vi "UHR-Fleezers Control (host) - Lorentz v4.vi"() -> ()   [LabVIEW 2014] (continued)
  in  "Chemyx Syringe Pump Serial Port":refnum<visa-resource-name>="ASRL3::INSTR"
  in  "Limit Min (MHz)":dbl=10.0 caption="Min (MHz)"
  in  "Limit Max (MHz)":dbl=16.0 caption="Max (MHz)"
  in  "Limits Enable":bool=TRUE caption="Enable"
  out "AI labels":string[](array[string])=["T1 Y", "T1 X", "T1 Sum", "T2 Y", "T2 X", "T2 Sum", "T1 FB X", "T1 FB Sum", "T2 FB X", "T2 FB Sum", "T3 Y", "T3 X", "T3 Sum", "PSD X", "PSD Y", "PSD Sum"]
  in  "Save Trap Pos. Data":bool=TRUE
  in  "Lower Ch. Cap.":bool
  in  "Top 3 Harvard Syringe Pump Serial Port":refnum<visa-resource-name>="Top-Pump3-COM4"
  out "Database link":path=path "C:/Home/Bustamante Lab/Comstock-LabView-Link.udl"
  out "connection reference":T25
  out "FPGA error out":errorcluster
  out "Trigger Signal":dbl[](graph)=[1.953852737276498, 1.8613052147403675]
  in  "Fish mask thresh":dbl=0.5
  in  "Normal (on) or masked test (off)":bool=TRUE
  in  "Stop F (pN) (mask)":dbl=1.0
  in  "Osc. freq. (Hz)":dbl=0.25
  in  "Trap shift\nmethod":bool=TRUE
  in  "Pause rotation":bool
  out "Waveform Chart":dbl(graph)
  in  "Trap 2 phase shift (deg)":dbl caption="Fixed phase shift (deg)"
  in  "Radius (MHz)":dbl=2.0 min=0.0 max=10.0 step=0.1
  out "Trap trajectories":cluster{dbl[], dbl[]}[](graph)
  in  "Move in a Circle":bool
  in  "Center Y Frequency (MHz)":dbl=31.0
  in  "Stop Moving":bool
  in  "2D Motion Frequency (Hz)":dbl=0.25
  in  "2D Motion Trap Separation (MHz)":dbl=0.75 caption="Fixed distance (MHz)" min=0.0 max=10.0 step=0.1
  in  "Time step (ms)":i64=10
  in  "N steps then stop":i32
  in  "Back to start on finish?":bool=TRUE
  in  "Counterclockwise/Clockwise":bool
  out "Trap 1 sum mean":dbl=nan format="%0.2f"
  out "Trap 2 sum mean":dbl=nan format="%0.2f"
  in  "index 1":i32=3
  in  "index 2":i32
  in  "test":bool
  in  "Reset graph":bool
  in  "N steps to plot":i32=1000
  out "Waveform Graph 2":waveform(dbl)(graph)
  in  "Offset 2":dbl
  in  "mult x":dbl
  in  "Offset":dbl
  out "N data samples":dbl
  out "Initial buffer time (s)":dbl
  in  "N initial buffer elements":u16=5000
  in  "Sound ON":bool
  in  "Carrier Frequency (Hz)":dbl=300.0
  in  "number of samples/ch":i32=100000
  in  "sample mode":T26=1 items=["Finite Samples", "Continuous Samples"]
  in  "device ID":u32
  in  "sound format":T27={"sample rate (S/s)"=22050.0, "number of channels"=2, "bits per sample"=16}
  in  "Volume":dbl=1.0 format="%0.2p"
  in  "interpolation mode":u16(ring)=1 items=["coerce", "linear", "spline", "FIR filter"]
  in  "tone or data":bool
  in  "Data channel to sound":i32
  in  "Base N trap periods":u32=50
  in  "Period scale factor":dbl=4.0
  in  "Trap osc amp (MHz)":dbl=1.0
  in  "Osc trap cont.":bool
  in  "Osc traps":bool
  out "Trap OSC Period (s)":dbl=0.003
  out "Writing waveform to fpga memory":bool
  in  "Save trap pos with cal":bool=TRUE
  in  "T1 Osc Enable":bool=TRUE
  in  "T2 Osc Enable":bool=TRUE
  out "DMA remainder":u64
  out "(total save/100) /osc period remainder":u32
  out "Total save/100 remainder":u32
  out "N osc/ (total save/100)":u64=25
  out "N osc / DMA":u64=100
  out "N trap osc periods per save":u64
  out "N trap osc periods per save remainder":u64
  in  "Command":string
  out "Reply":string
  in  "Send Command":bool
  out "Preamp Error Out":errorcluster
  in  "Gain Mode":string(combo)="0"
  in  "Invert Signal":bool
  in  "Sensitivity":string(combo)="0"
  in  "Offset Current Sign":bool=TRUE
  in  "Offset Current Value":string(combo)
  in  "Offset Current":bool
  in  "Bias Voltage":bool
  in  "Bias Voltage (mV)":i32
  in  "Filter Type":string(combo)="4"
  in  "Lowpass 3dB Point":string(combo)="6"
  in  "Highpass 3dB Point":string(combo)
  in  "Filter Reset":bool
  out "Command Sent":string
  out "Gain":string(combo)="0"
  out "Pressure":dbl=0.014364525990046895 format="%#.2f"
  in  "Vacuum":bool=TRUE
  in  "Set zero pressure":bool caption="Vent pressure"
  in  "DAQmx Device Name":tag="Lumicks"
  out "Channel 3":T28={"X Pos (mm)"=0.15566698, "Y Pos (mm)"=-0.21665113, "Z Pos (mm)"=-0.11814949} {"Y Pos (mm)" format="%.3f"; "Z Pos (mm)" format="%.3f"; "X Pos (mm)" format="%.3f"}
  out "Channel 2":T28={"X Pos (mm)"=0.39374417, "Y Pos (mm)"=-0.0075209886, "Z Pos (mm)"=-0.07494753} {"Y Pos (mm)" format="%.3f"; "Z Pos (mm)" format="%.3f"; "X Pos (mm)" format="%.3f"}
  out "Channel 1":T28={"X Pos (mm)"=-1.904501, "Y Pos (mm)"=-0.42059234, "Z Pos (mm)"=-0.07494753} {"Y Pos (mm)" format="%.3f"; "Z Pos (mm)" format="%.3f"; "X Pos (mm)" format="%.3f"}
  in  "Motor Cruise Param":T29={"Y Acc (mm/s^2)"=0.1, "Y Vmax (mm/s)"=1.0, "X Acc (mm/s^2)"=0.3, "X Vmax (mm/s)"=1.0, "Z Acc (mm/s^2)"=0.1, "Z Vmax (mm/s)"=0.1}
  out "Channel 4":T28={"X Pos (mm)"=-2.403743, "Y Pos (mm)"=0.10211637, "Z Pos (mm)"=-0.074918374} {"Y Pos (mm)" format="%.3f"; "Z Pos (mm)" format="%.3f"; "X Pos (mm)" format="%.3f"}
  out "0 Position":T28 {"Y Pos (mm)" format="%.3f"; "Z Pos (mm)" format="%.3f"; "X Pos (mm)" format="%.3f"}
  in  "Calibration Cruise Param":T29={"Y Acc (mm/s^2)"=2.0, "Y Vmax (mm/s)"=0.5, "X Acc (mm/s^2)"=2.0, "X Vmax (mm/s)"=0.5, "Z Acc (mm/s^2)"=0.1, "Z Vmax (mm/s)"=0.1}
  in  "Read Coordinates":bool
  in  "Write Coordinates":bool
  in  "4-Experiment position":bool
  in  "Capture Channel 4":bool
  out "Channel 5":T28={"X Pos (mm)"=0.15566698, "Y Pos (mm)"=-0.2807253, "Z Pos (mm)"=-0.118062034} {"Y Pos (mm)" format="%.3f"; "Z Pos (mm)" format="%.3f"; "X Pos (mm)" format="%.3f"}
  in  "Motor settings (Z)":cluster{"Vmax (mm/s)":sgl, "Acc (mm/s/s)":sgl}={"Vmax (mm/s)"=0.02, "Acc (mm/s/s)"=0.2}
  in  "Motor settings (X,Y)":cluster{"Vmax (mm/s)":sgl, "Acc (mm/s/s)":sgl}={"Vmax (mm/s)"=0.2, "Acc (mm/s/s)"=0.2}
  in  "Motor Limits":T30={"XMAX"=3.5, "XMIN"=-5.0, "YMAX"=2.0, "YMIN"=-2.0, "ZMAX"=2.0, "ZMIN"=-2.0}
  out "XYZ position":sgl[](array[numeric])=[0.3568097, 0.022271454, -0.22568797]
  in  "Go to 0 at stop?":bool
  in  "Write Coordinates path":path=path "C:/Data/Coordinates"
  in  "Read Coordinates path":path=path "C:/Data/Coordinates"
  in  "Capture Channel 3":bool
  in  "Capture Channel 2":bool
  in  "Capture Channel 1":bool
  in  "2-Get bead 2":bool
  in  "3-Calibration position":bool
  in  "1-Get bead 1":bool
  in  "MG17Motor Z":refnum<k7>(container)
  in  "MG17Motor Y":refnum<k7>(container)
  in  "MG17Motor X":refnum<k7>(container)
  in  "Motor Serial Numbers":cluster{"X":i32, "Y":i32, "Z":i32}={"X"=83829798, "Y"=83829822, "Z"=83829794}
  out "Distance to target":T31={"X  (mm)"=0.15566698, "Y  (mm)"=-0.2807253, "Z  (mm)"=-0.118062034} {"Y  (mm)" format="%.3f"; "Z  (mm)" format="%.3f"; "X  (mm)" format="%.3f"}
  out "Current position":T32={"X  Pos (mm)"=0.15566698, "Y Pos  (mm)"=-0.2807253, "Z Pos  (mm)"=-0.118062034} {"Y Pos  (mm)" format="%.3f"; "Z Pos  (mm)" format="%.3f"; "X  Pos (mm)" format="%.3f"}
  out "Motor Error Cluster out":errorcluster
  # "X"
  # "Y"
  # "Data Saving"
  # "External fluorescence triggering tests:"
  # "After"
  # "During"
  # "Trap On?"
  # "BD Flow ON?"
  # "Samp Flow ON?"
  # "Trap Trig. Fl.?"
  # "Zero It"
  # "Floor it\n(e.g., hp unwinding)"
  # "1"
  # "2"
  # "Fl. Down"
  # "Fl. Up"
  # "T1 Y"
  # "T1 X"
  # "T1 Sum"
  # "T2 Y"
  # "T2 X"
  # "T2 Sum"
  # "FB1 X"
  # "FB1 Sum"
  # "FB2 X"
  # "FB2 Sum"
  # "T3 Y"
  # "T3 X"
  # "T3 Sum"
  # "PSD X"
  # "PSD Y"
  # "PSD Sum"
  # "Trap Display:"
  # "APD Display:"
  # "DAQ"
  # "Trap Manipulation"
  # "Bead Calibration"
  # "MCL trap"
  # "Fine Motor Control"
  # "Bottom Pump (#1)"
  # "Central Sample Channels"
  # "Top Pump (#3)"
  # "Rate param is ul/h\nVolume param is ul"
  # "Chemyx Pump 2"
  # "Units: \n1 = ml/m\n2 = ml/h\n3 = ul/m\n4 = ul/h"
  # "Choose method of updating trap RF values: false is usual, true is use external loop method\n(in order to increase possible delay between X and Y signals -- to synchronize X and Y switching)"
  # "Delay to switch frequency and amplitude of boards.\nUsed to align phases of boards (finely)."
  # "X"
  # "Y"
  # "Oscillate Set 1 freq. (debugging)"
  # "BD 1"
  # "BD 2"
  # "Amp switch 1st is disabled in the fpga!\nSeems its also frequency that needs to go first (for all boards tested so far)."
  # "AOD Raster Scan"
  # "Approx. trap separations"
  # "X"
  # "Y"
  # "FPGA\nreading"
  # "DMA\ntransfer"
  # "APD Integration Loop"
  # "APD Gates"
  # "APD 2 (Cy5)"
  # "APD 3 (Cy2)"
  # "APD 1 (Cy3)"
  # "X"
  # "2D"
  # "Y"
  # "1D"
  # "Digital Out Control"
  # "Analog Out Control (Feedback Loop)"
  # "Laser Intensity Analog Input"
  # "Operational note:\n\nUse the digital out control to adjust red laser\ntiming (fine tuning).\n\nAt the moment, the red laser analog out\ncontrol timing is identical and set by green \nlaser AO timing (in the same loop).  Otherwise\nyou can not get synchronous timing with the\ncurrent AO expansion board.\n\nSimilarly, the AI measurement is also \nsimultaneous for all three lasers (for the same\nreason).\n\nThese controls are kept for possible future\nuse."
  # "Analog Out Control (Feedback Loop)"
  # "Digital Out Control"
  # "Laser Intensity Analog Input"
  # "Operational note:\n\nThe AI measurement is simultaneous for all three lasers\n(see red laser note).\n\nThese controls are kept for possible future use."
  # "Analog Out Control (Feedback Loop)"
  # "Laser Intensity Analog Input"
  # "Digital Out Control"
  # "Total AI Rates (NOT rates/trap)"
  # "(Samples/trap x Trap Sets)"
  # "(Samples/channel x\n8 if averaging (8 channels)\n4 if no averaging)"
  # "Trap 1"
  # "Trap 2"
  # "Flour./Trap 3"
  # "External Video Window"
  # "3: IR LED\n2: Blue LED"
  # "MCL Position Debugging"
  # "Temporary Control Storage\n(these used to be somewhere else, still want to keep them)"
  # "Database config"
  # "Y"
  # "X"
  # "Trap Position Difference Limits"
  # "Start trapping above center (> center MHz)\n\nNegative trap separation means trap 2 follows\n(starts to the right)"
  # "Initialization"
  # "Radius initially determined by center\nand current location (then can be changed)"
  # "Active (oscillating) trap calibration:"
  # "All these remainders\nshould be 0."
types:
  T1 = typedef "IMAQ Image.ctl" = refnum<image>
  T2 = cluster{"APD 1 Rate (Hz)":dbl, "APD 2 Rate (Hz)":dbl, "APD 3 Rate (Hz)":dbl, "Sigma/Mean 1":dbl, "Int Time (s)":dbl, "Sigma 1":dbl, "Sigma 2":dbl, "Sigma 3":dbl, "Sigma/Mean 2":dbl, "Sigma/Mean 3":dbl}
  T3 = enum32{"Actions", "Cal.", "Fish", "Force FB", "Fixed Traps", "Trig. Fl.", "Dipping", "Profile Flow", "Fluor. Yanking", "Stepping"}
  T4 = enum32{"Dual Display (Trap + Fluor.)", "Imaging", "Current Saved Data", "Display All", "FFT", "High Res Display"}
  T5 = cluster{"T1 X":dbl, "T2 X":dbl, "T3 X":dbl, "T3 Y":dbl}
  T6 = cluster{"T1 X":bool, "T2 X":bool, "T3 X":bool, "T3 Y":bool}
  T7 = enum32{"Status", "Sample Stage", "Syringe Pump", "Trap Control (RF)", "APD Counting", "Fluorescence Laser Control", "Trap AI", "Video", "FPGA", "Misc. Configuration", "Triggering", "2D Movement", "Sound Out", "Trap calibration", "Current Measurement", "Lumicks and motors"}
  T8 = cluster{"T2 alpha_x (nm/V)":dbl, "T2 offset_x (mV)":dbl, "T2 kappa_x (pN/nm)":dbl}
  T9 = cluster{"T1 alpha_x (nm/V)":dbl, "T1 offset_x (mV)":dbl, "T1 kappa_x (pN/nm)":dbl}
  T10 = cluster{"Pump 1":cluster{"Diameter (mm)":dbl, "Units":dbl, "Volume":dbl, "Rate":dbl}, "Pump 2":cluster{"Diameter (mm)":dbl, "Units":dbl, "Volume":dbl, "Rate":dbl}, "Pump 3":cluster{"Diameter (mm)":dbl, "Units":dbl, "Volume":dbl, "Rate":dbl}}
  T11 = enum32{"IR Laser Interlacing (Direct RF Board Control Method)", "AOD Raster Scan", "Feedback on Trap Intensity", "Feedback on Trap Position"}
  T12 = typedef "LVPoint32TypeDef.ctl" = cluster{"Horizontal":i32, "Vertical":i32}
  T13 = cluster{"Scan Range AOD (nm) 2":dbl, "Step Size AOD (nm) 2":dbl, "Scan Speed AOD (nm/s) 2":dbl, "Number of scans (AOD) 2":u16, "Label":string}[]
  T14 = cluster{"proportional gain (Kc)":i16, "integral gain (Kc*Ts/Ti)":i16, "derivative gain (Kc*Td/Ts)":i16}
  T15 = cluster{"Trap 1":fxp<+/-,16,1>, "Trap 2":fxp<+/-,16,1>}
  T16 = enum32{"Main Setting", "Details", "Dynamic FB settings", "Semi Passive Mode"}
  T17 = cluster{"proportional gain (Kc)":fxp<+/-,16,8>, "integral gain (Kc*Ts/Ti)":fxp<+/-,16,8>, "derivative gain (Kc*Td/Ts)":fxp<+/-,16,8>}
  T18 = cluster{"output high":fxp<+/-,16,1>, "output low":fxp<+/-,16,1>}
  T19 = cluster{"Set 1":fxp<+/-,16,1>, "Set 2":fxp<+/-,16,1>}
  T20 = cluster{"Trap 1X offset":dbl[], "Trap 2X offset":dbl[]}
  T21 = enum32{"Main Controls", "Green laser (532 nm)", "Red laser (633 nm)", "Blue laser (473 nm)"}
  T22 = cluster{"Set 1":bool, "Set 2":bool, "Set 3":bool}
  T23 = cluster{"baud rate":u32, "data bits":u16, "parity":enum16{"None", "Odd", "Even", "Mark", "Space"}, "stop bits":u16, "flow control":u16, "Time out (ms)":u32}
  T24 = typedef "LVMinMaxIncTypeDef.ctl" = cluster{"Minimum":dbl, "Maximum":dbl, "Increment":dbl}
  T25 = typedef "NI_Database_API.lvlib/Conn ObjectReference.ctl" = refnum<k1>
  T26 = typedef "Sampling Mode.ctl" = i32
  T27 = typedef "Sound Data Format.ctl" = cluster{"sample rate (S/s)":dbl, "number of channels":i32, "bits per sample":i32}
  T28 = cluster{"X Pos (mm)":sgl, "Y Pos (mm)":sgl, "Z Pos (mm)":sgl}
  T29 = cluster{"Y Acc (mm/s^2)":sgl, "Y Vmax (mm/s)":sgl, "X Acc (mm/s^2)":sgl, "X Vmax (mm/s)":sgl, "Z Acc (mm/s^2)":sgl, "Z Vmax (mm/s)":sgl}
  T30 = cluster{"XMAX":sgl, "XMIN":sgl, "YMAX":sgl, "YMIN":sgl, "ZMAX":sgl, "ZMIN":sgl}
  T31 = cluster{"X  (mm)":sgl, "Y  (mm)":sgl, "Z  (mm)":sgl}
  T32 = cluster{"X  Pos (mm)":sgl, "Y Pos  (mm)":sgl, "Z Pos  (mm)":sgl}
  T33 = typedef "nirio_resource_hc.ctl" = tag
  T34 = typedef "Image Type" = u32
  T35 = typedef "XDNodeRunTimeDep.lvlib/timing_clust.ctl" = cluster{"Expected End [f-1]":u64, "Actual End [f-1]":u64, "Finished Late? [f-1]":bool, "Expected End [i-1]":u64, "Actual End [i-1]":u64, "Finished Late? [i-1]":bool, "Expected Start [i]":u64, "Actual Start [i]":u64, "Expected Start [f]":u64, "Actual Start [f]":u64, "Source Name":string, "Structure Name":string, "Period":i64, "Deadline":i64, "Offset":i64, "Start":i64, "Priority":i32, "Timeout":i32, "Mode":T36, "Wakeup Reason":T37, "Error":errorcluster, "Source Type":string, "Secondary Source Type":string, "Global End Time":u64, "Global Start Time":u64, "Frame Duration":u64, "Iteration Duration":u64, "Assigned CPU":i32, "I/O Scan Engine Mode":u32}
  T36 = typedef "XDNodeRunTimeDep.lvlib/nitl_modes.ctl" = enum32{"No Change", "Process missed periods, maintain original phase", "Discard missed periods, maintain original phase", "Process missed periods, ignore original phase", "Discard missed periods, ignore original phase"}
  T37 = typedef "XDNodeRunTimeDep.lvlib/wakeup.ctl" = enum32{"Normal", "Aborted", "Asynchronous wakeup", "Timing source error", "Timed loop error", "Timeout"}
  T38 = enum16{"big-endian, network order", "native, host order", "little-endian"}
  T39 = enum16{"open", "replace", "create", "open or create", "replace or create", "replace or create with confirmation"}
  T40 = cluster{"X axis":i32, "Y axis":i32, "Z axis":i32, "X axis rotation":i32, "Y axis rotation":i32, "Z axis rotation":i32, "U axis":i32, "V axis":i32}
  T41 = cluster{"button 1":bool, "button 2":bool, "button 3":bool, "button 4":bool, "button 5":bool, "button 6":bool, "button 7":bool, "button 8":bool, "button 9":bool, "button 10":bool, "button 11":bool, "button 12":bool, "button 13":bool, "button 14":bool, "button 15":bool, "button 16":bool, "button 17":bool, "button 18":bool, "button 19":bool, "button 20":bool, "button 21":bool, "button 22":bool, "button 23":bool, "button 24":bool, "button 25":bool, "button 26":bool, "button 27":bool, "button 28":bool, "button 29":bool, "button 30":bool, "button 31":bool, "button 32":bool}
  T42 = cluster{"[0]":sgl, "[1]":sgl, "[2]":sgl, "[3]":sgl, "[4]":sgl, "[5]":sgl, "[6]":sgl, "[7]":sgl, "[8]":sgl, "[9]":sgl, "[10]":sgl, "[11]":sgl, "[12]":sgl, "[13]":sgl, "[14]":sgl}
  T43 = typedef "IMAQdx.ctl" = refnum<k21>
  T44 = typedef "Pressure Control.lvclass/Pressure Control Config.ctl" = cluster{"daqmx_channel":string, "terminal_configuration":string}
  T45 = cluster{string, "TTL line # Pressure Up":u8, bool, bool}
  T46 = cluster{string, "TTL line # Pressure Down":u8, bool, bool}
  T47 = cluster{string, "TTL line # Pressure Vacuum":u8, bool, bool}
  T48 = cluster{string, "TTL line # Pressure Vacuum":u8, bool, bool}[]
  T49 = cluster{"New Image":T1, "New Image":T1, "New Image":T1, "New Image":T1, "New Image":T1}
  T50 = typedef "openfpgaref.8.6.ctl" = refnum<k20>
  T51 = enum32{"Status", "Sample Stage", "Syringe Pump", "Trap Control (RF)", "APD Counting", "Fluorescence Laser Control", "Trap AI", "Video", "FPGA"}
  T52 = enum32{"Status", "Sample Stage", "Syringe Pump", "Trap Control (RF)", "APD Counting", "Fluorescence Laser Control", "Trap AI", "Video", "FPGA", "Misc. Configuration"}
  T53 = enum16{"CONNECT", "INITIALIZE VALVES", "DISCONNECT", "MOVE VALVE"}
  T54 = enum16{"empty", "write", "read oldest (queue)", "read newest (stack)", "read all"}
  T55 = cluster{"Scan Range AOD (nm) 2":dbl, "Step Size AOD (nm) 2":dbl, "Scan Speed AOD (nm/s) 2":dbl, "Number of scans (AOD) 2":u16, "Label":string}
  T56 = cluster{"[0]":dbl, "[1]":dbl, "[2]":dbl, "[3]":dbl, "[4]":dbl, "[5]":dbl}
  T57 = cluster{"Diameter (mm)":dbl, "Units":dbl, "Volume":dbl, "Rate":dbl}
  T58 = cluster{"Left":i32, "Top":i32, "Width":u32, "Height":u32}
  T59 = cluster{cluster{"Left":i32, "Top":i32, "Width":u32, "Height":u32}}[]
  T60 = typedef "Sound Output Task ID.ctl" = u32
  T61 = enum32{"Normal Display", "Dual Display (APD)", "FFT", "High Res Display"}
  T62 = cluster{"Origin Pixel":cluster{"X":sgl, "Y":sgl}, "Angle Relative to Horizontal (deg)":sgl, "Axis Reference":u32}
  T63 = typedef "Simple Grid Descriptor" = cluster{"X Step":sgl, "Y Step":sgl, "Unit":T64}
  T64 = typedef "Image Unit" = enum32{"Undefined", "Angström", "Micrometer", "Millimeter", "Centimeter", "Meter", "Kilometer", "Microinch", "Inch", "Feet", "Nautical miles", "Standard miles", "Steps"}
  T65 = cluster{"averaging mode":u16, "weighting mode":u16, "number of averages":u32}
  T66 = cluster{"dB On (F)":bool, "unwrap phase (F)":bool, "convert to degree (F)":bool}
  T67 = cluster{"Scan Range (nm)":dbl, "MCL Step Position Ratio":dbl, "MCL/AOM Scale Tweak":dbl, "MCL X Cal (nm/V)":dbl, "MCL Step Increment (V_int)":dbl, "Total Counts (ticks)":u16, "Scan steps (AOD)":u64, "Cycles/step (AOD)":u64}
  T68 = cluster{"Actual MCL Inc (V)":dbl, "Scan steps (MCL)":u64, "Scan lines (y)":u64, "AO1":dbl, "AO2":dbl}
  T69 = cluster{"APD 1":u32[], "APD 2":u32[], "APD 3":u32[]}
  T70 = cluster{"RMS[0]":dbl, "RMS[1]":dbl, "RMS[2]":dbl, "RMS[3]":dbl}
  T71 = cluster{"Mean [0]":dbl, "Mean [1]":dbl, "Mean [2]":dbl, "Mean [3]":dbl}
  T72 = cluster{"f0":dbl, "df":dbl, "magnitude":dbl[]}[][]
  T73 = cluster{"Comment (data description)":string, "Channel 1 Buffer":string, "Channel 2 Buffer":string, "Channel 3 Buffer":string, "Title":string, "DNA Construct":string, "Bead diameter":dbl, "Name":string}
diagram:
  w25 = 90.0
  w53 = T34 2 items=["Grayscale (U8)", "Grayscale (I16)", "Grayscale (SGL)", "Complex (CSG)", "RGB (U32)", "HSL (U32)", "RGB (U64)", "Grayscale (U16)"] ("Image Type")
  # "If no error continue shutdown of motors\nas planned. If there is an error - DO NOT \ntry to shut down motors."
  # "Thorlabs motor control and camera feed added by Ronen"
  # "X limits"
  # "Amp Lmits"
  # "Freq Limits"
  # "Changed by Ronen - All events relating to activation of the pumps have been disabled: 56, 55, 54, 53, 52, 51, 50, 49, 48, 47, 46, 45, 44, 43, 41, 40"
  # "Harvard Pump control disabled by Hendrik"
  # "Settings to help prevent AOM/D damage"
  # "Initialize the FPGA DAQ card itself"
  # "Reset the DAQ card."
  # "Specify the DAQ card and the FPGA code to run"
  # "Bottom 1 Harvard"
  # "Top 3 Harvard"
  # "Center Harvard"
  n1 = Cluster To Array(cluster="Motor Serial Numbers") -> (array=w3:i32[])
  n2 = call <vilib>:"Query Input Devices.vi"() -> ("error out"=w13:errorcluster)  [unwired: 8 in, 3 out]
  n3 = call <vilib>:"Initialize Joystick.vi"("error in (no error)"=w13, "device index"=1) -> ("error out"=w10:errorcluster, "device ID"=w11:refnum<k1>)  [unwired: 8 in]
  n4 = call "initializemotors.vi"("Motor serial numbers"=w3, "MG17Motor Z"="MG17Motor Z", "MG17Motor Y"="MG17Motor Y", "MG17 Motor X"="MG17Motor X") -> ("Output errors"=w1:errorcluster[], "Output references"=w14:refnum<k7>[])  [unwired: 6 in]
  n5 = while {
    tunnel: w14 -> [w109]
    shift-right: [w99] -> w5
    shift-left: _ -> [w108]
    tunnel: w11 -> [w107]
    shift-right: [w98] -> w9
    shift-left: w10 -> [w106]
    tunnel: [w105] -> w8
    shift-right: [w100] -> w7
    shift-left: _ -> [w104]
    tunnel: w3 -> [w102]
    stop <- w101 stop-if-true
    n6 = event shown="[5] \"1-Get bead 1\": Value Change" {
      selector: _ -> [_ _ _ _ _ _ _ _ _ _ _ _]
      dyn-events: _ -> [_ _ _ _ _ _ _ _ _ _ _ _]
      timeout: 50 -> [_ _ _ _ _ _ _ _ _ _ _ _]
      tunnel: w109 -> [w114 w128 w134 w141 w147 w151 w180 w209 w238 w265 _ _]
      tunnel: [_ w129 w130 w137 w143 w149 w178 w207 w236 w266 w282 w334] -> w99
      tunnel: w108 -> [_ w126 w133 w139 w146 w150 w179 w208 w237 w267 w276 w337]
      tunnel: [_ _ _ _ _ _ _ _ _ TRUE _ _] -> w101
      tunnel: w107 -> [w123 _ _ _ _ _ _ _ _ _ _ _]
      tunnel: w106 -> [w122 _ _ _ _ _ _ _ _ _ _ _]
      tunnel: [w121 _ _ _ _ _ _ _ _ _ _ _] -> w98
      tunnel: [w120 _ _ _ _ _ _ _ _ _ _ _] -> w105
      tunnel: [w116 _ _ _ _ _ _ _ _ _ _ _] -> w100
      tunnel: w104 -> [_ _ _ _ _ _ _ _ _ _ _ _]
      tunnel: w102 -> [w110 _ _ _ _ w148 w177 w206 w235 _ _ _]
      event Timeout {
        n7 = event-data() -> ()  [unwired: 1 in, 3 out]
        n8 = call-poly <vilib>:"Acquire Input Data.vi"("device ID"=w123, "error in (no error)"=w122) -> ("device ID"=w120:refnum<k1>, "axis info"=w118:T40, "button info"=w119:T41, "error out"=w121:errorcluster)  [unwired: 13 in, 1 out]
        n9 = call "motor XY setMeng.vi"("Motor settings Z"="Motor settings (Z)", "Motor serial numbers"=w110, "Motor settings (X,Y)"="Motor settings (X,Y)", "Array 2"=w114) -> ("Array 3"=w115:errorcluster[])  [unwired: 6 in, 1 out]
        n10 = call "motorJoystickcore.vi"("button info"=w119, "axis info"=w118, "error in"=w115, "Motor Limits"="Motor Limits", "Array in"=w114, "Motor serial numbers"=w110) -> ("error out"=w116:errorcluster[], "XYZ position"=→"XYZ position":sgl[])  [unwired: 4 in]
      }
      event "Capture Channel 1": Mouse Down {
        n11 = event-data() -> ()  [unwired: 1 in, 7 out]
        n12 = control-ref of="Channel 1"() -> (w127:refnum<vi>)
        n13 = call "captureTopBottomExp.vi"("error in (no error)"=w126, "Array in"=w128, "Cluster in"=w127) -> ("error out"=w125:errorcluster, "Value"=w124:T28)  [unwired: 7 in]
        n14 = property on="Channel 1" class="Clust (strict)"(error in=w125, "Value"=w124) -> (error out=w129:errorcluster)  [unwired: 1 in, 1 out]
      }
      event "Capture Channel 2": Mouse Down {
        n15 = event-data() -> ()  [unwired: 1 in, 7 out]
        n16 = control-ref of="Channel 2"() -> (w135:refnum<vi>)
        n17 = call "captureTopBottomExp.vi"("error in (no error)"=w133, "Array in"=w134, "Cluster in"=w135) -> ("error out"=w131:errorcluster, "Value"=w132:T28)  [unwired: 7 in]
        n18 = property on="Channel 2" class="Clust (strict)"(error in=w131, "Value"=w132) -> (error out=w130:errorcluster)  [unwired: 1 in, 1 out]
      }
      event "Capture Channel 3": Mouse Down {
        n19 = event-data() -> ()  [unwired: 1 in, 8 out]
        n20 = control-ref of="Channel 3"() -> (w140:refnum<vi>)
        n21 = call "captureTopBottomExp.vi"("error in (no error)"=w139, "Array in"=w141, "Cluster in"=w140) -> ("error out"=w138:errorcluster, "Value"=w136:T28)  [unwired: 7 in]
        n22 = property on="Channel 3" class="Clust (strict)"(error in=w138, "Value"=w136) -> (error out=w137:errorcluster)  [unwired: 1 in, 1 out]
      }
      event "Capture Channel 4": Mouse Down {
        n23 = event-data() -> ()  [unwired: 1 in, 8 out]
        n24 = control-ref of="Channel 4"() -> (w145:refnum<vi>)
        n25 = call "captureTopBottomExp.vi"("error in (no error)"=w146, "Array in"=w147, "Cluster in"=w145) -> ("error out"=w144:errorcluster, "Value"=w142:T28)  [unwired: 7 in]
        n26 = property on="Channel 4" class="Clust (strict)"(error in=w144, "Value"=w142) -> (error out=w143:errorcluster)  [unwired: 1 in, 1 out]
      }
      event "1-Get bead 1": Value Change {
        n27 = event-data() -> ()  [unwired: 1 in, 6 out]
        n28 = flat-sequence {
          tunnel: w151 -> [w156]
          tunnel: w150 -> [w155]
          tunnel: w148 -> [w153]
          tunnel: [w154] -> w149
          frame #0 {
            n29 = node-c288(50) -> (w159:T35)  [unwired: 5 in]
            n30 = timed-loop {
              timing: w159 -> [_]
              timing-out: [_] -> w158
              tunnel: w156 -> [w167]
              tunnel: w155 -> [w169]
              tunnel: [w163] -> w154
              tunnel: w153 -> [_]
              stop <- w162 stop-if-true
              n31 = node-c288() -> ()  [unwired: 1 in, 1 out]
              n32 = control-ref of="Current position"() -> (w170:refnum<vi>)
              n33 = control-ref of="Motor Cruise Param"() -> (w166:refnum<vi>)
              n34 = local read "Channel 1"() -> (w160:T28)
              n35 = call "captureTopBottomExp.vi"("error in (no error)"=w169, "Array in"=w167, "Cluster in"=w170) -> ("error out"=w168:errorcluster, "Value"=w161:T28)  [unwired: 7 in]
              n36 = property on="Current position" class="Clust (strict)"(error in=w168, "Val(Sgnl)"=w161) -> (error out=w164:errorcluster)  [unwired: 1 in, 1 out]
              n37 = call "Test_distance_to_position.vi"("Channel"=w160, "Current position"=w161) -> ("All out of range?"=w162:bool, "Output distance"=w165:T28)
              n38 = call "gotoTopBotExp2Ronen.vi"("error in (no error)"=w164, "Distance to target"=w165, "motor setting"=w166, "Array of all references"=w167) -> ("error out"=w163:errorcluster)  [unwired: 7 in]
              n39 = node-c288() -> ()  [unwired: 1 in, 1 out]
            }
            n40 = local write "1-Get bead 1"(FALSE ("Value (Signaling)")) -> ()
            n41 = node-c288(w158) -> ()  [unwired: 1 out]
          }
        }
      }
      event "2-Get bead 2": Value Change {
        n42 = event-data() -> ()  [unwired: 1 in, 6 out]
        n43 = flat-sequence {
          tunnel: w180 -> [w185]
          tunnel: w179 -> [w184]
          tunnel: w177 -> [w182]
          tunnel: [w183] -> w178
          frame #0 {
            n44 = node-c288(50) -> (w188:T35)  [unwired: 5 in]
            n45 = timed-loop {
              timing: w188 -> [_]
              timing-out: [_] -> w187
              tunnel: w185 -> [w196]
              tunnel: w184 -> [w198]
              tunnel: [w192] -> w183
              tunnel: w182 -> [_]
              stop <- w191 stop-if-true
              n46 = node-c288() -> ()  [unwired: 1 in, 1 out]
              n47 = control-ref of="Current position"() -> (w199:refnum<vi>)
              n48 = control-ref of="Motor Cruise Param"() -> (w195:refnum<vi>)
              n49 = local read "Channel 2"() -> (w189:T28)
              n50 = call "captureTopBottomExp.vi"("error in (no error)"=w198, "Array in"=w196, "Cluster in"=w199) -> ("error out"=w197:errorcluster, "Value"=w190:T28)  [unwired: 7 in]
              n51 = property on="Current position" class="Clust (strict)"(error in=w197, "Val(Sgnl)"=w190) -> (error out=w193:errorcluster)  [unwired: 1 in, 1 out]
              n52 = call "Test_distance_to_position.vi"("Channel"=w189, "Current position"=w190) -> ("All out of range?"=w191:bool, "Output distance"=w194:T28)
              n53 = call "gotoTopBotExp2Ronen.vi"("error in (no error)"=w193, "Distance to target"=w194, "motor setting"=w195, "Array of all references"=w196) -> ("error out"=w192:errorcluster)  [unwired: 7 in]
              n54 = node-c288() -> ()  [unwired: 1 in, 1 out]
            }
            n55 = local write "2-Get bead 2"(FALSE ("Value (Signaling)")) -> ()
            n56 = node-c288(w187) -> ()  [unwired: 1 out]
          }
        }
      }
      event "3-Calibration position": Value Change {
        n57 = event-data() -> ()  [unwired: 1 in, 6 out]
        n58 = flat-sequence {
          tunnel: w209 -> [w214]
          tunnel: w208 -> [w213]
          tunnel: w206 -> [w211]
          tunnel: [w212] -> w207
          frame #0 {
            n59 = node-c288(50) -> (w217:T35)  [unwired: 5 in]
            n60 = timed-loop {
              timing: w217 -> [_]
              timing-out: [_] -> w216
              tunnel: w214 -> [w225]
              tunnel: w213 -> [w227]
              tunnel: [w221] -> w212
              tunnel: w211 -> [_]
              stop <- w220 stop-if-true
              n61 = node-c288() -> ()  [unwired: 1 in, 1 out]
              n62 = control-ref of="Current position"() -> (w228:refnum<vi>)
              n63 = control-ref of="Motor Cruise Param"() -> (w224:refnum<vi>)
              n64 = local read "Channel 3"() -> (w218:T28)
              n65 = call "captureTopBottomExp.vi"("error in (no error)"=w227, "Array in"=w225, "Cluster in"=w228) -> ("error out"=w226:errorcluster, "Value"=w219:T28)  [unwired: 7 in]
              n66 = property on="Current position" class="Clust (strict)"(error in=w226, "Val(Sgnl)"=w219) -> (error out=w222:errorcluster)  [unwired: 1 in, 1 out]
              n67 = call "Test_distance_to_position.vi"("Channel"=w218, "Current position"=w219) -> ("All out of range?"=w220:bool, "Output distance"=w223:T28)
              n68 = call "gotoTopBotExp2Ronen.vi"("error in (no error)"=w222, "Distance to target"=w223, "motor setting"=w224, "Array of all references"=w225) -> ("error out"=w221:errorcluster)  [unwired: 7 in]
              n69 = node-c288() -> ()  [unwired: 1 in, 1 out]
            }
            n70 = local write "3-Calibration position"(FALSE ("Value (Signaling)")) -> ()
            n71 = node-c288(w216) -> ()  [unwired: 1 out]
          }
        }
      }
      event "4-Experiment position": Value Change {
        n72 = event-data() -> ()  [unwired: 1 in, 6 out]
        n73 = flat-sequence {
          tunnel: w238 -> [w243]
          tunnel: w237 -> [w242]
          tunnel: w235 -> [w240]
          tunnel: [w241] -> w236
          frame #0 {
            n74 = node-c288(50) -> (w246:T35)  [unwired: 5 in]
            n75 = timed-loop {
              timing: w246 -> [_]
              timing-out: [_] -> w245
              tunnel: w243 -> [w254]
              tunnel: w242 -> [w256]
              tunnel: [w250] -> w241
              tunnel: w240 -> [_]
              stop <- w249 stop-if-true
              n76 = node-c288() -> ()  [unwired: 1 in, 1 out]
              n77 = control-ref of="Current position"() -> (w257:refnum<vi>)
              n78 = control-ref of="Motor Cruise Param"() -> (w253:refnum<vi>)
              n79 = local read "Channel 4"() -> (w247:T28)
              n80 = call "captureTopBottomExp.vi"("error in (no error)"=w256, "Array in"=w254, "Cluster in"=w257) -> ("error out"=w255:errorcluster, "Value"=w248:T28)  [unwired: 7 in]
              n81 = property on="Current position" class="Clust (strict)"(error in=w255, "Val(Sgnl)"=w248) -> (error out=w251:errorcluster)  [unwired: 1 in, 1 out]
              n82 = call "Test_distance_to_position.vi"("Channel"=w247, "Current position"=w248) -> ("All out of range?"=w249:bool, "Output distance"=w252:T28)
              n83 = call "gotoTopBotExp2Ronen.vi"("error in (no error)"=w251, "Distance to target"=w252, "motor setting"=w253, "Array of all references"=w254) -> ("error out"=w250:errorcluster)  [unwired: 7 in]
              n84 = node-c288() -> ()  [unwired: 1 in, 1 out]
            }
            n85 = local write "4-Experiment position"(FALSE ("Value (Signaling)")) -> ()
            n86 = node-c288(w245) -> ()  [unwired: 1 out]
          }
        }
      }
      event "Stop All": Value Change {
        n87 = event-data() -> ()  [unwired: 1 in, 6 out]
        n88 = case shown="True" "Go to 0 at stop?" {
          tunnel: w267 -> [_ w272]
          tunnel: [_ w271] -> w266
          tunnel: w265 -> [_ w270]
          frame False {
          }
          frame True {
            n89 = control-ref of="Motor Cruise Param"() -> (w269:refnum<vi>)
            n90 = control-ref of="0 Position"() -> (w273:refnum<vi>)
            n91 = call "gotoTopBotExp2.vi"("error in (no error)"=w272, "position"=w273, "motor setting"=w269, "appended array"=w270) -> ("error out"=w271:errorcluster)  [unwired: 7 in]
          }
        }
      }
      event "Write Coordinates": Value Change {
        # "Writes coordinates to file"
        n92 = event-data() -> ()  [unwired: 1 in, 6 out]
        n93 = local write "Write Coordinates"(FALSE ("Value (Signaling)")) -> ()
        n94 = property on="Channel 3" class="Clust (strict)"() -> ("Value"=w279:T28)  [unwired: 2 in, 2 out]
        n95 = property on="Channel 5" class="Clust (strict)"() -> ("Value"=w277:T28)  [unwired: 2 in, 2 out]
        n96 = property on="Channel 4" class="Clust (strict)"() -> ("Value"=w278:T28)  [unwired: 2 in, 2 out]
        n97 = property on="Channel 1" class="Clust (strict)"() -> ("Value"=w281:T28)  [unwired: 2 in, 2 out]
        n98 = property on="Channel 2" class="Clust (strict)"() -> ("Value"=w280:T28)  [unwired: 2 in, 2 out]
        n99 = Unbundle By Name(w281) -> ("X Pos (mm)"=w305:sgl, "Y Pos (mm)"=w304:sgl, "Z Pos (mm)"=w303:sgl)
        n100 = Unbundle By Name(w280) -> ("X Pos (mm)"=w302:sgl, "Y Pos (mm)"=w301:sgl, "Z Pos (mm)"=w300:sgl)
        n101 = Unbundle By Name(w279) -> ("X Pos (mm)"=w299:sgl, "Y Pos (mm)"=w298:sgl, "Z Pos (mm)"=w297:sgl)
        n102 = Unbundle By Name(w278) -> ("X Pos (mm)"=w296:sgl, "Y Pos (mm)"=w295:sgl, "Z Pos (mm)"=w294:sgl)
        n103 = Unbundle By Name(w277) -> ("X Pos (mm)"=w293:sgl, "Y Pos (mm)"=w292:sgl, "Z Pos (mm)"=w291:sgl)
        n104 = Build Array(w305, w304, w303, w302, w301, w300, w299, w298, w297, w296, w295, w294, w293, w292, w291) -> (w287:sgl[])
        n105 = Open/Create/Replace File(file path (use dialog)="Write Coordinates path", error in=w276, operation (0:open)=T39."replace or create", access (0:read/write)=enum16{"read/write", "read-only", "write-only"}."read/write") -> (refnum out=w288:refnum<file>, error out=w285:errorcluster)  [unwired: 2 in, 1 out]
        n106 = Write to Binary File(file (use dialog)=w288, data=w287, error in=w285, 9:T38."big-endian, network order" ("byte order (0:big-endian, network order)")) -> (refnum out=w286:refnum<file>, error out=w284:errorcluster)  [unwired: 2 in, 1 out]
        n107 = Close File(refnum=w286, error in=w284) -> (error out=w282:errorcluster)  [unwired: 1 out]
      }
      event "Read Coordinates": Value Change {
        # "Reads coordinates from file"
        n108 = event-data() -> ()  [unwired: 1 in, 6 out]
        n109 = local write "Read Coordinates"(FALSE ("Value (Signaling)")) -> ()
        n110 = Open/Create/Replace File(file path (use dialog)="Read Coordinates path", error in=w337) -> (refnum out=w340:refnum<file>, error out=w341:errorcluster)  [unwired: 4 in, 1 out]
        n111 = Read from Binary File(5:sgl[] [], 8:w341, 11:w340) -> (0:w335:errorcluster, 2:w333:sgl[], 3:w336:refnum<file>)  [unwired: 3 in, 1 out]
        n112 = Close File(refnum=w336, error in=w335) -> (error out=w334:errorcluster)  [unwired: 1 out]
        n113 = local read "Channel 5"() -> (w327:T28)
        n114 = local read "Channel 4"() -> (w328:T28)
        n115 = local read "Channel 2"() -> (w330:T28)
